vi "FPGA_SCTLTest1.vi"() -> ()   [LabVIEW 2014]
uses:
  <vilib>/rvi/Emulation/niFpgaGetClockAttributes.vi
  <vilib>/rvi/Emulation/niFpgaSctlEmulationGetInTimedLoop.vi
  <vilib>/rvi/Emulation/niFpgaEmulationReportErrorSimple.vi
  <vilib>/rvi/Emulation/niFpgaCriticalErrorInLSC.vi
panel:
  out "Sorted Array":i16[](array[numeric])
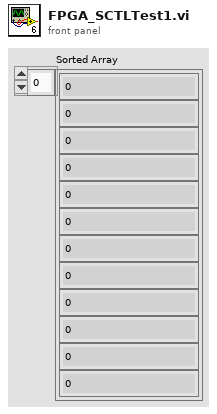
[diagram p1: front panel]
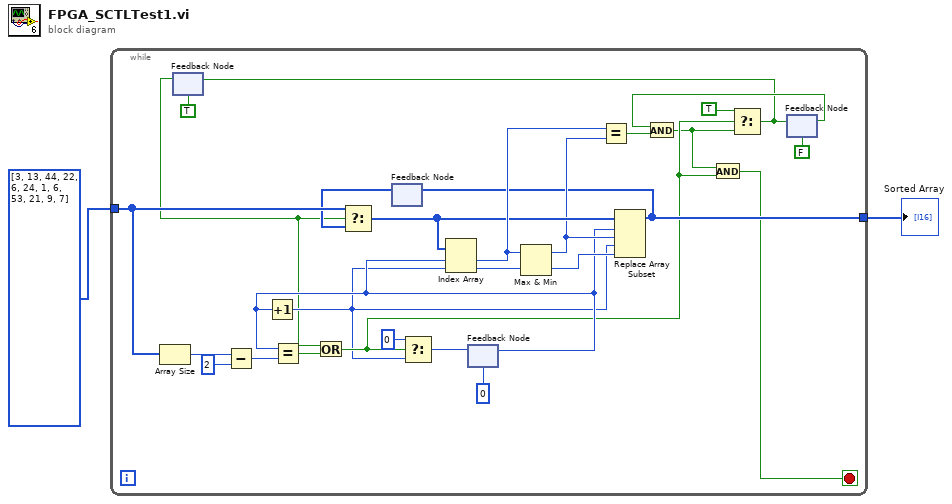
[diagram p0: block diagram]
diagram:
  n1 = while {
    tunnel: i16[] [3, 13, 44, 22, 6, 24, 1, 6, 53, 21, 9, 7] -> [w29]
    tunnel: [w15] -> w1
    stop <- w4 stop-if-true
    n2 = Array Size(array=w29) -> (size(s)=w28:i32)
    n3 = feedback #1(TRUE) -> (w6:bool)
    n4 = Subtract(x=w28, y=2) -> (x-y=w26:i32)
    n5 = feedback #2() -> (w14:i16[])  [unwired: 1 in]
    n6 = Select(t=w29, s=w6, f=w14) -> (s? t:f=w22:i16[])
    n7 = feedback #3(0 ("y")) -> (w16:i32)
    n8 = Increment(x=w16) -> (x+1=w7:i32)
    n9 = Equal?(x=w16, y=w26) -> (x = y?=w25:bool)
    n10 = Or(x=w6, y=w25) -> (x .or. y?=w9:bool)
    n11 = Select(t=0 ("y"), s=w9, f=w7) -> (s? t:f=w18:i32)
    n12 = Index Array(array=w22, index #1=w16, index #2=w7) -> (element #1=w23:i16, element #2=w24:i16)
    n13 = feedback-in #3(w18) -> ()
    n14 = Max & Min(x=w23, y=w24) -> (max(x,y)=w21:i16, min(x,y)=w20:i16)
    n15 = Equal?(x=w23, y=w21) -> (x = y?=w13:bool)
    n16 = Replace Array Subset(array=w22, new element #1=w21, index #1=w16, new element #2=w20, index #2=w7) -> (w15:i16[])
    n17 = feedback-in #2(w15) -> ()
    n18 = feedback #4(FALSE ("t")) -> (w10:bool)
    n19 = And(x=w10, y=w13) -> (x .and. y?=w8:bool)
    n20 = And(x=w8, y=w9) -> (x .and. y?=w4:bool)
    n21 = Select(t=TRUE, s=w9, f=w8) -> (s? t:f=w3:bool)
    n22 = feedback-in #1(w3) -> ()
    n23 = feedback-in #4(w3) -> ()
  }
  "Sorted Array" <- w1
